vi "postMessage.vi"(8 "error in (no error)":errorcluster, 11 "postMessageCluster":T1) -> (0 "error out":errorcluster)   [LabVIEW 2013, in "SlackinLabViewLib.lvlib"]
uses:
  <vilib>/httpClient/ClientHandle.ctl
  Controls/postMessageCluster.ctl
  <vilib>/httpClient/POSTBuffer.vi
  SlackinLabViewLib.lvlib
  <vilib>/httpClient/LabVIEWHTTPClient.lvlib
panel:
  out "client handle out":T2
  out "headers":string
  out "body":string
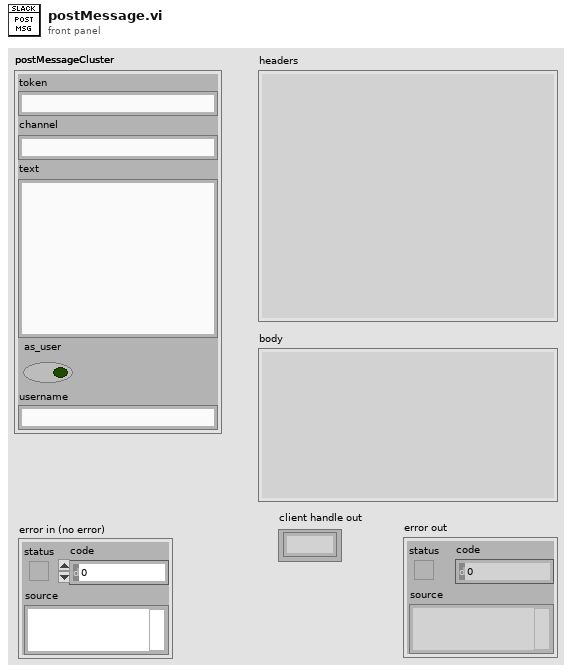
[diagram p1: front panel]
types:
  T1 = typedef "postMessageCluster.ctl" = cluster{"token":string, "channel":string, "text":string, "as_user":bool, "username":string}
  T2 = typedef "LabVIEWHTTPClient.lvlib/ClientHandle.ctl" = refnum<k1>
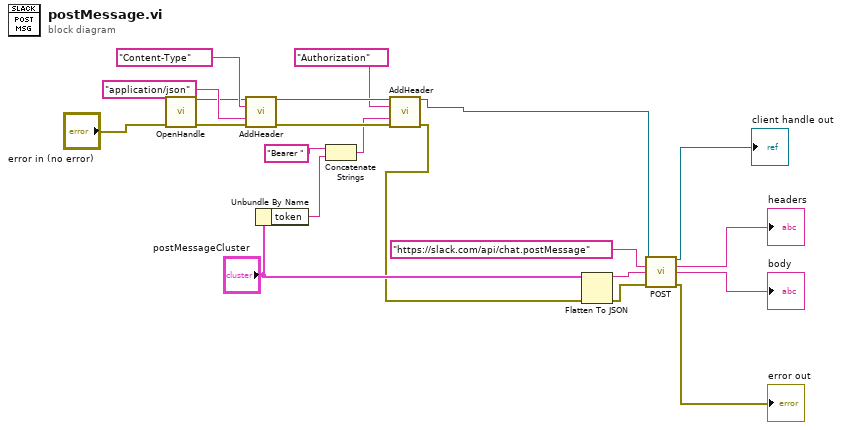
[diagram p0: block diagram]
diagram:
  n1 = call <vilib>:"OpenHandle.vi"("error in (no error)"="error in (no error)") -> ("client handle out"=w12:T2, "error out"=w8:errorcluster)  [unwired: 13 in]
  n2 = call <vilib>:"AddHeader.vi"("client handle"=w12, "header"="Content-Type", "value"="application/json", "error in (no error)"=w8) -> ("client handle out"=w10:T2, "error out"=w9:errorcluster)  [unwired: 10 in]
  n3 = Unbundle By Name("postMessageCluster") -> ("token"=w4:string)
  n4 = Concatenate Strings("Bearer " ("string"), w4) -> (w6:string)
  n5 = call <vilib>:"AddHeader.vi"("client handle"=w10, "header"="Authorization", "value"=w6, "error in (no error)"=w9) -> ("client handle out"=w11:T2, "error out"=w2:errorcluster)  [unwired: 10 in]
  n6 = Flatten To JSON(anything="postMessageCluster", error in (no error)=w2) -> (JSON string=w16:string, 11:w15:errorcluster)  [unwired: 1 in]
  n7 = call-poly <vilib>:"POST.vi"("client handle"=w11, "url"="https://slack.com/api/chat.postMessage", "buffer"=w16, "error in (no error)"=w15) -> ("client handle out"=→"client handle out":T2, "headers"=→"headers":string, "body"=→"body":string, "error out"=→"error out":errorcluster)  [unwired: 8 in]
